vi "更新数据.vi"(8 "error in (no error)":errorcluster caption="错误输入（无错误）", 10 "采集数据":dbl[](array[numeric]), 11 "数据存储 输入":refnum<class "数据存储.lvclass"> caption="DNL_LabVIEW Object in") -> (0 "error out":errorcluster caption="错误输出", 3 "数据存储 输出":refnum<class "数据存储.lvclass"> caption="DNL_LabVIEW Object out")   [LabVIEW 2013, in "数据存储.lvclass"]
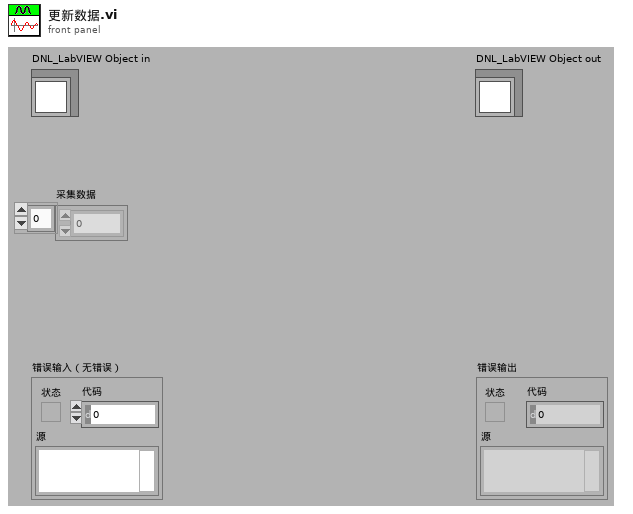
[diagram p1: front panel]
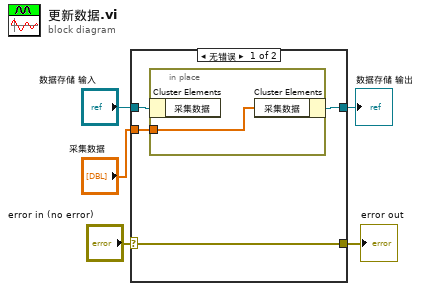
[diagram p0: block diagram]
diagram:
  n1 = case shown="无错误" "error in (no error)" {
    selector: "error in (no error)" -> [w9 w12]
    tunnel: [w9 w12] -> w4
    tunnel: "数据存储 输入" -> [w8 w11]
    tunnel: "采集数据" -> [w7 _]
    tunnel: [w6 w11] -> w1
    frame No Error {
      n2 = in-place {
        in-place-border: w7 -> [w10]
        n3 = in-place-cluster #1(w8) -> ()  [unwired: 1 out]
        n4 = in-place-cluster #1("采集数据"=w10) -> (w6:refnum<class "数据存储.lvclass">)
      }
    }
    frame Error {
    }
  }
  "error out" <- w4
  "数据存储 输出" <- w1
